vi "LVFunction_Imop_HasoSetupFile_GetInformation.vi"(0 "WFS_setup_file IN":path, 11 "error in (no error)":errorcluster) -> (4 "WFS_setup_file OUT":path, 6 "HASO specifications":T1, 8 "SoftwareOptionsList":string[](array[string]), 10 "SDKOptionsList":string[](array[string]), 15 "error out":errorcluster)   [LabVIEW 2020]
uses:
  Controls/HasoSpecifications.ctl
  Controls/General dimensions definition.ctl
  Controls/Point2D.ctl
  Controls/Point2Df.ctl
panel:
  out "InternalOptionsList":string[](array[string])
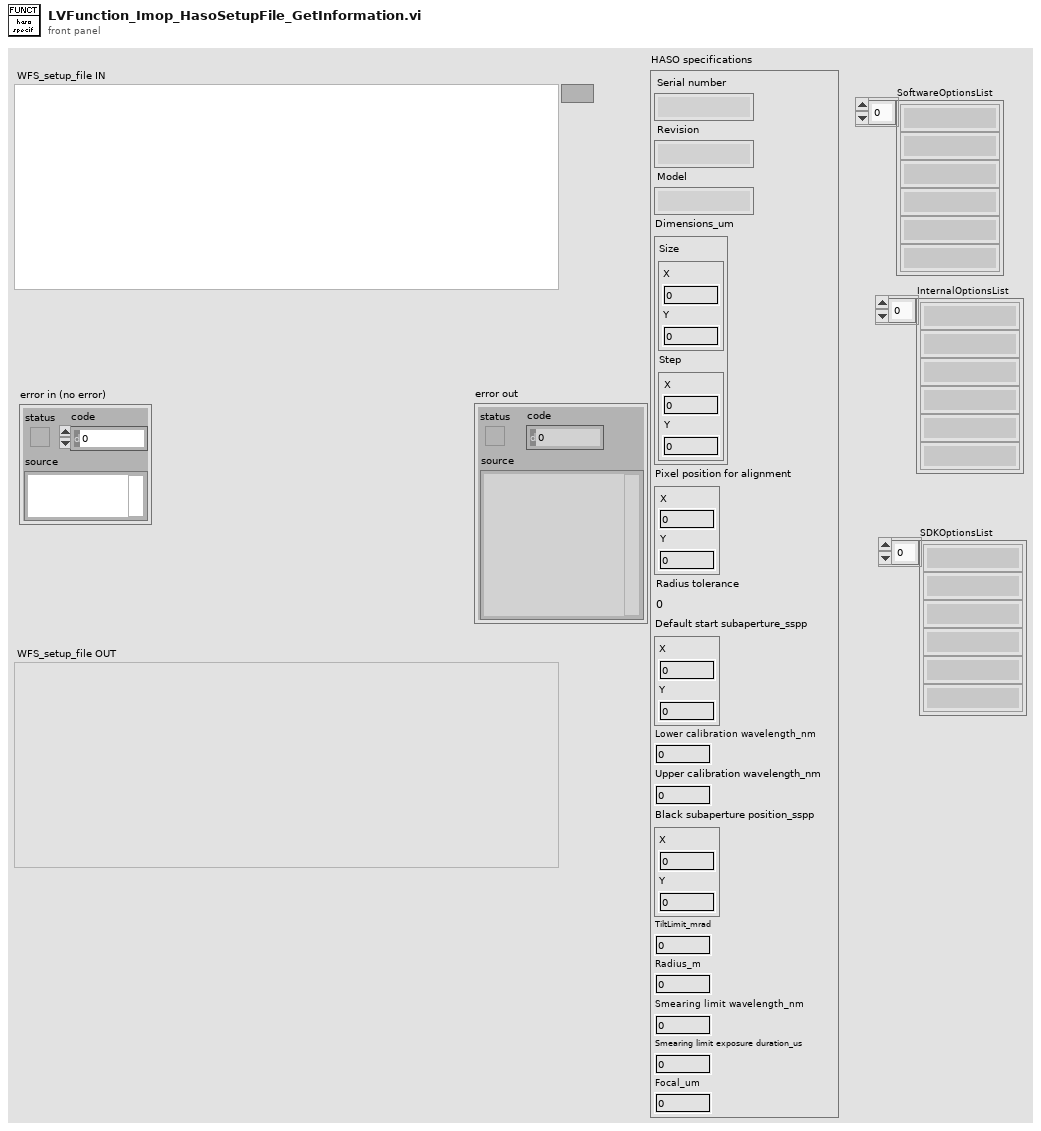
[diagram p1: front panel]
types:
  T1 = typedef "HasoSpecifications.ctl" = cluster{"Serial number":string, "Revision":string, "Model":string, "Dimensions_um":T2, "Pixel position for alignment":T4, "Radius tolerance":u16, "Default start subaperture_sspp":T3, "Lower calibration wavelength_nm":dbl, "Upper calibration wavelength_nm":dbl, "Black subaperture position_sspp":T3, "TiltLimit_mrad":dbl, "Radius_m":dbl, "Smearing limit wavelength_nm":dbl, "Smearing limit exposure duration_us":dbl, "Focal_um":dbl}
  T2 = typedef "General dimensions definition.ctl" = cluster{"Size":T3, "Step":T4}
  T3 = typedef "Point2D.ctl" = cluster{"X":u32, "Y":u32}
  T4 = typedef "Point2Df.ctl" = cluster{"X":sgl, "Y":sgl}
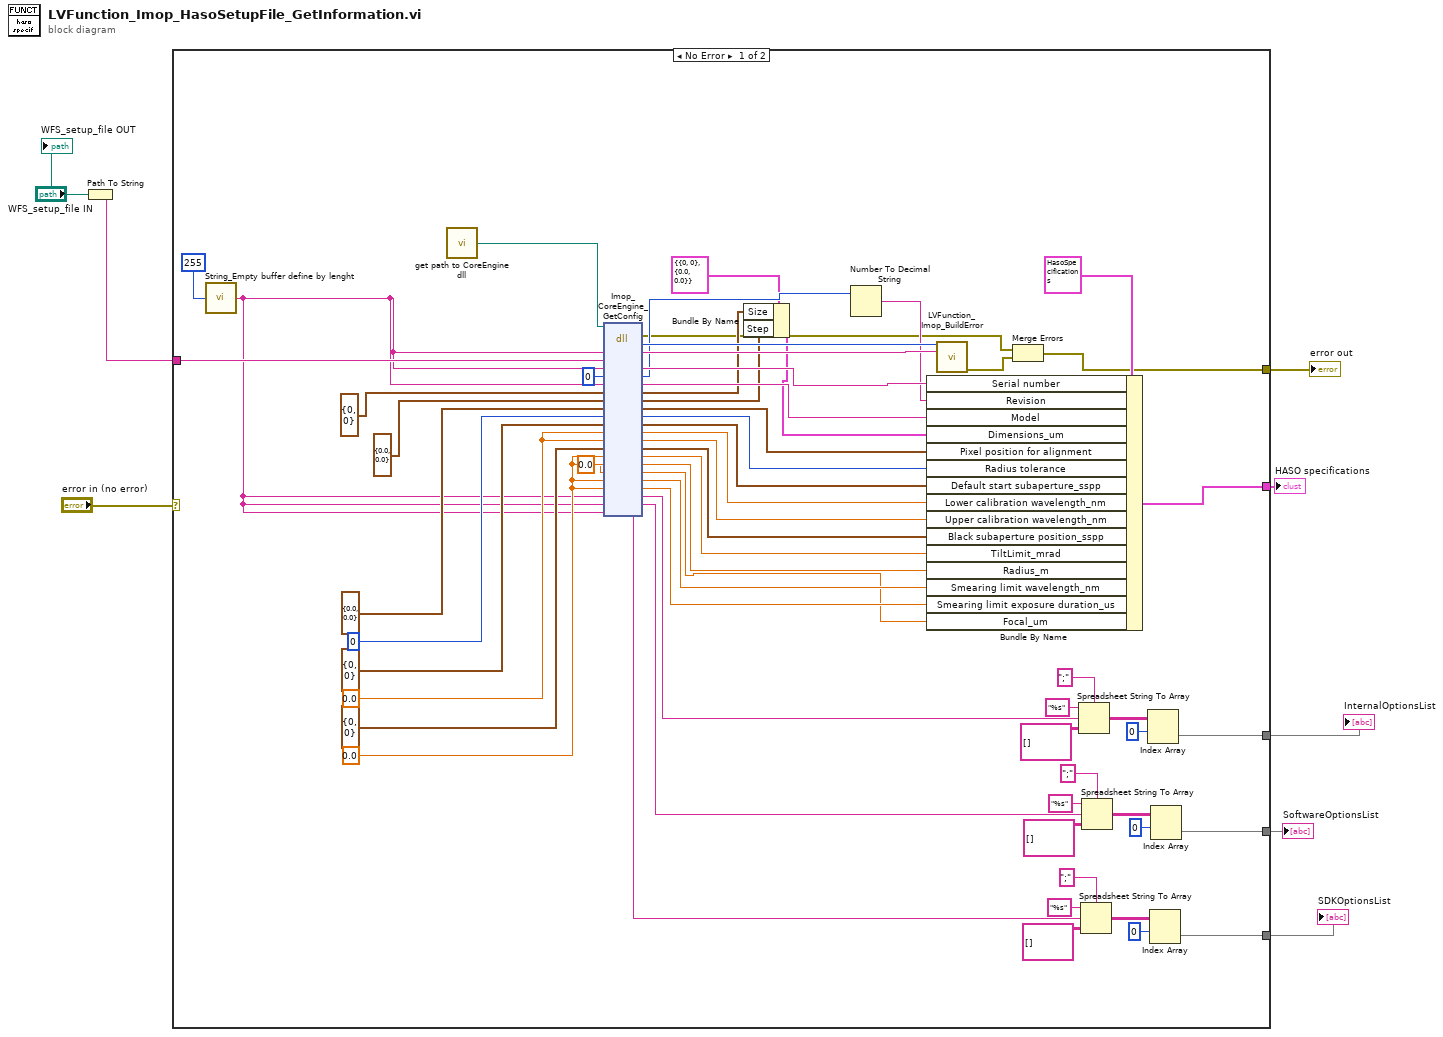
[diagram p0: block diagram]
diagram:
  n1 = Path To String(path="WFS_setup_file IN") -> (string=w6:string)
  n2 = case shown="No Error" "error in (no error)" {
    selector: "error in (no error)" -> [_ w70]
    tunnel: [w9 w70] -> w7
    tunnel: w6 -> [w49 _]
    tunnel: [w42 _] -> w4
    tunnel: [w51 _] -> w5
    tunnel: [w33 _] -> w3
    tunnel: [w12 _] -> w2
    frame No Error {
      w61 = 0.0 ("LowerCalibrationWavelength_nm")
      w63 = 0.0 ("LowerCalibrationWavelength_nm")
      n3 = call "String_Empty buffer define by lenght.vi"("Lenght (255)"=255 ("dimension size")) -> ("Empty buffer"=w14:string)
      n4 = call "get path to CoreEngine dll.vi"() -> ("path to wavekit library"=w68:path)  [unwired: 14 in, 1 out]
      n5 = dll-call lib="D:/SOFTware/HASO_v3/SVN_trunk/ImOpCoreEngine4_LV2011/DLLs/ImopEngine4_vc100d.dll" fn="Imop_CoreEngine_GetConfig"(path in=w68, "message"=w14, "config_file_path"=w49, "SerialNumber"=w14, "revision"=u32 0, "model"=w14, "nb_subapertures"=T3 {"X"=0, "Y"=0} ("Size"), "ulens_step_um"=T4 {"X"=0.0, "Y"=0.0} ("Step"), "PositionForAlignment_pixels"=T4 {"X"=0.0, "Y"=0.0} ("Pixel position for alignment"), "RadiusTolerance_pixels"=0, "DefaultStartSubaperture_sspp"=T3 {"X"=0, "Y"=0} ("Default start subaperture_sspp"), "LowerCalibrationWavelength_nm"=w63, "UpperCalibrationWavelength_nm"=w63, "BlackSubaperturePosition_sspp"=T3 {"X"=0, "Y"=0} ("Default start subaperture_sspp"), "TiltLimit_mrad"=w61, "Radius_m"=w61, "micro_lens_focal"=0.0, "SmearingLimitWavelength_nm"=w61, "SmearingLimitExposureDuration_S"=w61, "InternalOptionsList"=w14, "SoftwareInfoList"=w14, "SdkInfoList"=w14) -> (error out=w11:errorcluster, "return type"=w69:i32, "message"=w48:string, "SerialNumber"=w47:string, "revision"=w30:u32, "model"=w32:string, "nb_subapertures"=w23:T3, "ulens_step_um"=w22:T4, "PositionForAlignment_pixels"=w60:T4, "RadiusTolerance_pixels"=w20:u16, "DefaultStartSubaperture_sspp"=w59:T3, "LowerCalibrationWavelength_nm"=w58:dbl, "UpperCalibrationWavelength_nm"=w57:dbl, "BlackSubaperturePosition_sspp"=w56:T3, "TiltLimit_mrad"=w55:dbl, "Radius_m"=w54:dbl, "micro_lens_focal"=w27:dbl, "SmearingLimitWavelength_nm"=w53:dbl, "SmearingLimitExposureDuration_S"=w52:dbl, "InternalOptionsList"=w34:string, "SoftwareInfoList"=w40:string, "SdkInfoList"=w13:string)  [unwired: 3 in, 1 out]
      n6 = Bundle By Name(cluster=T2 {"Size"={"X"=0, "Y"=0}, "Step"={"X"=0.0, "Y"=0.0}} ("Dimensions"), "Size"=w23, "Step"=w22) -> (w21:T2)
      n7 = Number To Decimal String(number=w30) -> (decimal integer string=w29:string)  [unwired: 1 in]
      n8 = Bundle By Name(cluster=T1 {"Serial number"="", "Revision"="", "Model"="", "Dimensions_um"={"Size"={"X"=0, "Y"=0}, "Step"={"X"=0.0, "Y"=0.0}}, "Pixel position for alignment"={"X"=0.0, "Y"=0.0}, "Radius tolerance"=0, "Default start subaperture_sspp"={"X"=0, "Y"=0}, "Lower calibration wavelength_nm"=0.0, "Upper calibration wavelength_nm"=0.0, "Black subaperture position_sspp"={"X"=0, "Y"=0}, "TiltLimit_mrad"=0.0, "Radius_m"=0.0, "Smearing limit wavelength_nm"=0.0, "Smearing limit exposure duration_us"=0.0, "Focal_um"=0.0} ("HASO specifications"), "Serial number"=w47, "Revision"=w29, "Model"=w32, "Dimensions_um"=w21, "Pixel position for alignment"=w60, "Radius tolerance"=w20, "Default start subaperture_sspp"=w59, "Lower calibration wavelength_nm"=w58, "Upper calibration wavelength_nm"=w57, "Black subaperture position_sspp"=w56, "TiltLimit_mrad"=w55, "Radius_m"=w54, "Smearing limit wavelength_nm"=w53, "Smearing limit exposure duration_us"=w52, "Focal_um"=w27) -> (w51:T1)
      n9 = call "LVFunction_Imop_BuildError.vi"("code"=w69, "String to Prepend to source (\"\")"=w48) -> ("error out"=w10:errorcluster)  [unwired: 13 in]
      n10 = Merge Errors(w11, w10) -> (w9:errorcluster)
      n11 = Spreadsheet String To Array(delimiter (Tab)=";", format string="%s", spreadsheet string=w34, array type (2D Dbl)=string[][] []) -> (array=w38:string[][])
      n12 = Spreadsheet String To Array(delimiter (Tab)=";", format string="%s", spreadsheet string=w13, array type (2D Dbl)=string[][] []) -> (array=w18:string[][])
      n13 = Spreadsheet String To Array(delimiter (Tab)=";", format string="%s", spreadsheet string=w40, array type (2D Dbl)=string[][] []) -> (array=w43:string[][])
      n14 = Index Array(array=w38, index (row)=0) -> (element=w33:string[])  [unwired: 1 in]
      n15 = Index Array(array=w18, index (row)=0) -> (element=w12:string[])  [unwired: 1 in]
      n16 = Index Array(array=w43, index (row)=0) -> (element=w42:string[])  [unwired: 1 in]
    }
    frame Error {
    }
  }
  "error out" <- w7
  "SoftwareOptionsList" <- w4
  "HASO specifications" <- w5
  "InternalOptionsList" <- w3
  "SDKOptionsList" <- w2
  "WFS_setup_file OUT" <- "WFS_setup_file IN"
